vi "GetData.vi"(0 "AlazarCluster":T13, 1 "Digitizer Settings":T9={"Digitizer delay (us) "=0.0, "rf points per line"=2048, "lines per plane"=128, "Samp Rate (Hz)"=100000000.0, "Additional dig delay (us)"=0.0, "Voltage Scale"=0.4, "Pre-Looks"=0, "Offset delay (us)"=0.0, "bits A/D"=8, "Avg Num"=1, "DigTimeOut"=5.0, "Rel Dig Delay"=0.0, "Dig Ch"=0, "LeCroyCluster"={"LeCroy Channels"=[TRUE, FALSE, FALSE, FALSE], "LC read pt offset"=0.0, "Sweep Avg"=FALSE}, "Main Digitizer"=enum."NI Digitizer", "Dig Config"=enum."Single channel", "Digitizer ID Cluster"={"Acqiris/Alazar/SP ID"=[], "NI Instr Handles"=[], "LeCroy VISA"="", "GaGe Handle"={"Handle"=0, "Sample size"=0, "Resolution"=0, "Offset"=0, "Channels"=0, "Boards"=0}, "ATS Ref"="ATS9350", "Acqiris Address"=["PCI::INSTR0"], "ADQRef"=refnum, "adq_cu_ptr"=refnum}, "Trigger Settings"={"Trig Source"=1, "Trig Coupling"=0, "Trig Slope"=0, "Level (mV)"=1500.0}, "Bulk Acq"=FALSE, "Bulk Start Indexes"=[], "Data Ref RF"=refnum, "NI ID/Channel"=[], "Total Dig CH"=1, "Xtra Ann Trig delay (us)"=10.0, "Fix Z Delay?"=FALSE, "One Way Transmission?"=FALSE, "Data Ref Log"=refnum} {"Trigger Settings"."Trig Slope" items=["Positive", "Negative"]; "Trigger Settings"."Level (mV)" format="%.2f"; "Trigger Settings"."Trig Coupling" items=["DC 1 MOhm", "AC 1 MOhm", "DC 50 Ohm", "AC 50 Ohm"]; "Trigger Settings"."Trig Source" items=["Chan 1", "External"]; "Rel Dig Delay" format="%.2f"; "DigTimeOut" format="%.2f"; "Avg Num" min=1; "Offset delay (us)" format="%.2f"; "Additional dig delay (us)" format="%.2f"; "Digitizer delay (us)" format="%.2f"}, 2 "Ann Array Params":T2={"Synth Foc?"=FALSE, "Focal Zones"=41, "Switch T/R"=0, "Trans Geometry (mm)"={"Transducer"=0, "Geo Focus"=12.0, "a (radius)"=3.0, "# of rings"=5, "kerf space "=0.1, "Center Freq"=12.0}, "Sub Ap Excite?"=FALSE, "Full Array Scan?"=FALSE, "Xmt/Rcv"={"XMIT"=[TRUE, TRUE, TRUE, TRUE, TRUE], "RCV"=[TRUE, TRUE, TRUE, TRUE, TRUE]}, "PulseSpacing (us)"=0.0, "Xmit Ring"=0, "XMIT CHS"=0, "RCV CHS"=0, "GPU?"=FALSE, "Save TIFF?"=FALSE, "downfactor"=1, "RCV 1CH"=0} {"RCV 1CH" items=["All", "1", "2", "3", "4", "5"]; "Trans Geometry (mm)"."Transducer" items=["6D 12R 40 MHz"=0, "10D 31R 20 MHz"=1, "10D 23R 20 MHz"=2, "6D 23R 40 MHz"=3, "4.5D 10.7R 40 MHz"=4, "9D 23.5R 20 MHz"=5, "9D 25.8R 20MHz"=6, "Enter"=99]; "Switch T/R" min=1 max=5 step=1}, 3 "Motion Settings":T5={"No Motion?"=FALSE, "Motion System"=enum."NI 735x", "Motion Bd ID"=1, "Motion Profile"="SMAC1", "# Axis"=1, "Reverse Z axis?"=TRUE, "SMAC Axis"=0, "scan pair"=enum."y-(x) scan", "RT fps"=6.0, "Steps per mm"=[1000, 1000, 1000, 1000], "Motor Parameters"={"velocity ct/s"=[10000.0, 10000.0, 10000.0, 50000.0], "accel ct/s^2"=[50000.0, 50000.0, 50000.0, 200000.0]}, "One Way Scan"=FALSE, "Reverse One Way Scan"=FALSE, "Global Position (mm)"=[], "Plane"=0, "Distance between\nscan lines (um)"=0.0, "Distance between\nscan planes (um)"=0.0, "number of scan planes"=1, "Total steps in line"=0, "Xtra plane\ndistance  (um)"=100, "Xtra planes "=1, "Add Axis"=FALSE, "overshoot cts"=200, "BKPT Shift"=0, "Scan Start Time (ms)"=0, "ESP VISA"="GPIB::1::INSTR", "3rd Axis"=1, "GL Ref Out"=refnum, "Galil Address"=""} {"3rd Axis" items=["x", "y", "z", "w"]; "Xtra planes" min=1; "Xtra plane\ndistance  (um)" min=0; "Distance between\nscan planes (um)" format="%.2f"; "Distance between\nscan lines (um)" format="%.2f"; "SMAC Axis" items=["None"=0, "Axis 1"=1, "Axis 2"=2, "Axis 3"=3, "Axis 4"=4, "Axis 5"=5, "Axis 6"=6, "Axis 7"=7, "Axis 8"=8, "Vector Space 1"=17, "Vector Space 2"=18, "Vector Space 3"=19, "Vector Space 4"=20]; "Motion Bd ID" min=1 max=32 step=1}, 4 "All files":string[](array[string]), 5 "error in":errorcluster, 6 "lines per plane mod":i32, 7 "Type of scan":T1, 8 "save?":bool=TRUE, 10 "Start Record":i32, 11 "Reverse ?":bool) -> (12 "Gain Array":T14(array[cluster]), 15 "Raw data out":i16[][][](array[numeric]), 19 "error out":errorcluster)   [LabVIEW 2022 SP3]
uses:
  Digitizers/-DigitizerRoutines/DigitizerSettings.ctl
  Digitizers/-DigitizerRoutines/Digitizer.ctl
  Digitizers/-DigitizerRoutines/DigConfig.ctl
  Digitizers/-DigitizerRoutines/DigitizerID.ctl
  C:/Windows/System32/ADQAPI_dotNet_helper.dll
  Motion Controllers/NI_controller/-NI_MotionRoutines/MotionParameters.ctl
  Motion Controllers/NI_controller/-NI_MotionRoutines/MotionSys.ctl
  Motion Controllers/-MotionRoutines/ScanAxis.ctl
  Motion Controllers/-MotionRoutines/3rdAxis.ctl
  Annular Array/-AnnularRoutines/AnnularArray.ctl
  Annular Array/-AnnularRoutines/TransGeometry.ctl
  Annular Array/-AnnularRoutines/ArrayGeometry.ctl
  Controls/ScanType2.ctl
  Pulsers/PulserGlobals.vi
  Motion Controllers/-MotionRoutines/MotionGlobals.vi
  Digitizers/Acqiris/-AcqirisRoutines/GetAcqSeq.vi
panel:
  # "1-D and 2-D B scan settings"
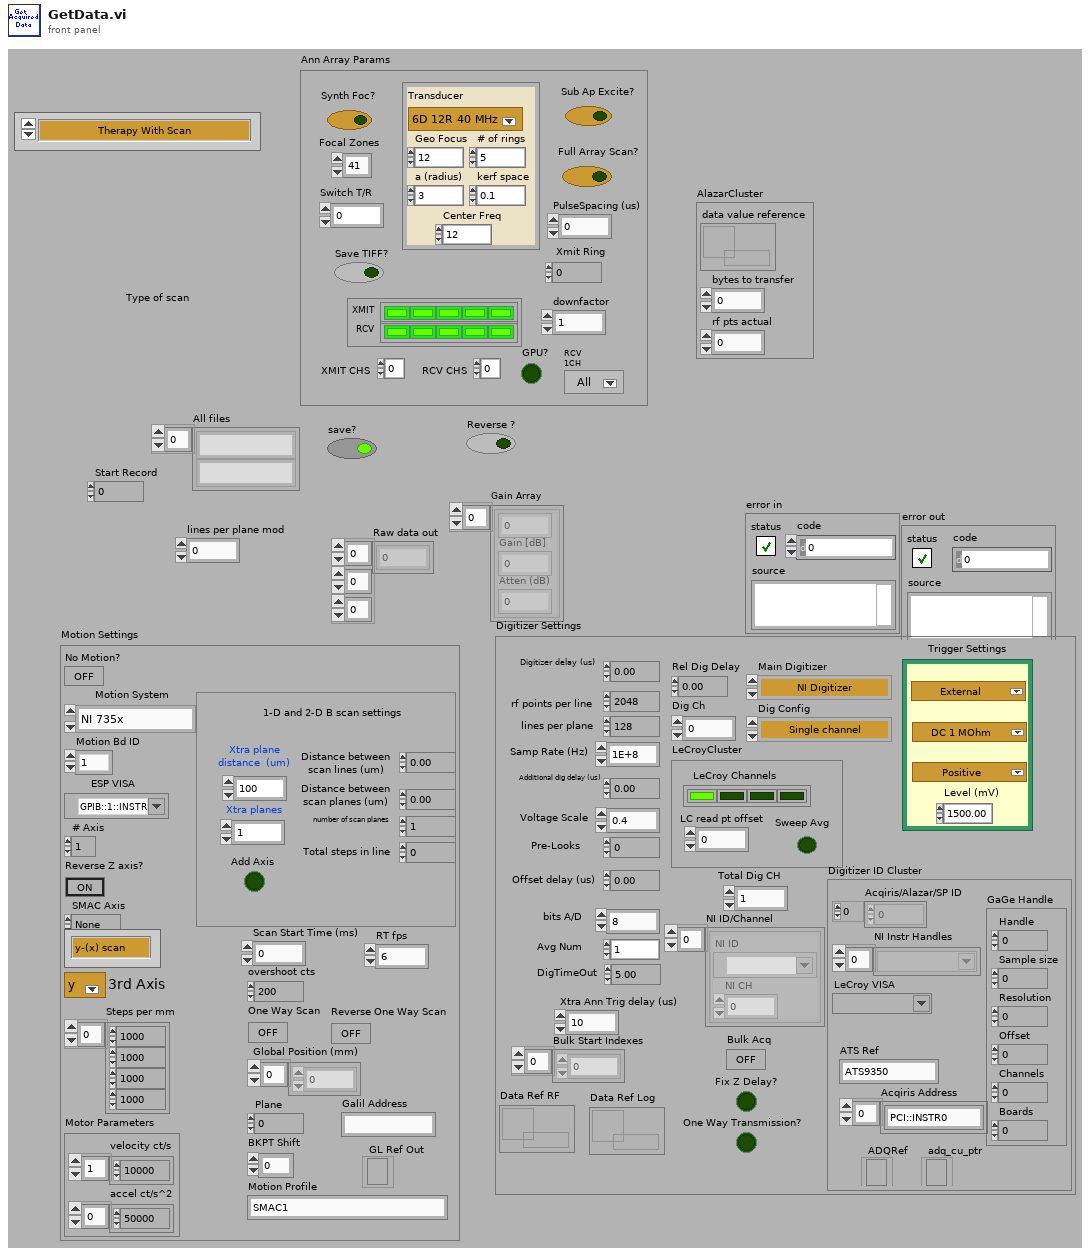
[diagram p1: front panel]
types:
  T1 = typedef "ScanType2.ctl" = enum16{"Therapy With Scan", "M scan", "M Scan With Therapy Burst", "1-D B Scan", "1-D B Scan With Therapy Burst", "2-D B Scan", "2-D B Scan With Therapy Burst", "Rotational Scan", "1-D B-Scan PRF", "2-D B-Scan PRF", "Real-Time Scan", "Contrast Agents", "1-D w/ Real-Time Set Up", "Dual Transducer", "Acoustic Microscopy", "Hydrophone Scanning"}
  T2 = typedef "AnnularArray.ctl" = cluster{"Synth Foc?":bool, "Focal Zones":i16, "Switch T/R":i16, "Trans Geometry (mm)":T3, "Sub Ap Excite?":bool, "Full Array Scan?":bool, "Xmt/Rcv":cluster{"XMIT":bool[], "RCV":bool[]}, "PulseSpacing (us)":sgl, "Xmit Ring":i32, "XMIT CHS":u8, "RCV CHS":u8, "GPU?":bool, "Save TIFF?":bool, "downfactor":i32, "RCV 1CH":u16}
  T3 = typedef "TransGeometry.ctl" = cluster{"Transducer":T4, "Geo Focus":dbl, "a (radius)":dbl, "# of rings":i32, "kerf space ":dbl, "Center Freq":dbl}
  T4 = typedef "ArrayGeometry.ctl" = u16
  T5 = typedef "MotionParameters.ctl" = cluster{"No Motion?":bool, "Motion System":T6, "Motion Bd ID":u8, "Motion Profile":string, "# Axis":i8, "Reverse Z axis?":bool, "SMAC Axis":u16, "scan pair":T7, "RT fps":sgl, "Steps per mm":i32[], "Motor Parameters":cluster{"velocity ct/s":dbl[], "accel ct/s^2":dbl[]}, "One Way Scan":bool, "Reverse One Way Scan":bool, "Global Position (mm)":dbl[], "Plane":i32, "Distance between\nscan lines (um)":sgl, "Distance between\nscan planes (um)":sgl, "number of scan planes":i32, "Total steps in line":i32, "Xtra plane\ndistance  (um)":i32, "Xtra planes ":i32, "Add Axis":bool, "overshoot cts":i32, "BKPT Shift":i32, "Scan Start Time (ms)":u32, "ESP VISA":refnum<visa-resource-name>, "3rd Axis":T8, "GL Ref Out":refnum<k7>, "Galil Address":string}
  T6 = typedef "MotionSys.ctl" = enum16{"MM3000", "NI 735x", "Newport ESP", "No Motion Card", "Galil"}
  T7 = typedef "ScanAxis.ctl" = enum16{"y-(x) scan", "x-(y) scan", "z-(x) scan", "z-(y) scan", "y-(z) scan", "x-(z) scan", "w-(x) scan", "w-(y) scan", "w-(z) scan", "x-(w) scan", "y-(w) scan", "z-(w) scan"}
  T8 = typedef "3rdAxis.ctl" = u16
  T9 = typedef "DigitizerSettings.ctl" = cluster{"Digitizer delay (us) ":dbl, "rf points per line":i32, "lines per plane":i32, "Samp Rate (Hz)":dbl, "Additional dig delay (us)":dbl, "Voltage Scale":dbl, "Pre-Looks":i32, "Offset delay (us)":dbl, "bits A/D":i8, "Avg Num":i32, "DigTimeOut":sgl, "Rel Dig Delay":sgl, "Dig Ch":i32, "LeCroyCluster":cluster{"LeCroy Channels":bool[], "LC read pt offset":dbl, "Sweep Avg":bool}, "Main Digitizer":T10, "Dig Config":T11, "Digitizer ID Cluster":T12, "Trigger Settings":cluster{"Trig Source":u16, "Trig Coupling":u16, "Trig Slope":u16, "Level (mV)":dbl}, "Bulk Acq":bool, "Bulk Start Indexes":i32[], "Data Ref RF":refnum<data-value>, "NI ID/Channel":cluster{"NI ID":refnum<k15>, "NI CH":i32}[], "Total Dig CH":i32, "Xtra Ann Trig delay (us)":dbl, "Fix Z Delay?":bool, "One Way Transmission?":bool, "Data Ref Log":refnum<data-value>}
  T10 = typedef "Digitizer.ctl" = enum16{"Acqiris Digitizer", "NI Digitizer", "LeCroy", "GaGe", "AlazarTech", "No Digitizer", "Teledyne"}
  T11 = typedef "DigConfig.ctl" = enum16{"Single channel", "2 Chans w/ 2 Acqiris", "2 Chans w/ 1 Acqiris", "5-CH Pulser New", "5-CH pulser w/ ann array", "5-pass style ann array", "Empty"}
  T12 = typedef "DigitizerID.ctl" = cluster{"Acqiris/Alazar/SP ID":u32[], "NI Instr Handles":refnum<k15>[], "LeCroy VISA":refnum<visa-resource-name>, "GaGe Handle":cluster{"Handle":u32, "Sample size":u32, "Resolution":i32, "Offset":i32, "Channels":u32, "Boards":u32}, "ATS Ref":string, "Acqiris Address":string[], "ADQRef":refnum<k24>, "adq_cu_ptr":refnum<k24>}
  T13 = cluster{"data value reference":refnum<data-value>, "bytes to transfer":u32, "rf pts actual":u32}
  T14 = cluster{sgl, "Gain [dB]  ":sgl, "Atten (dB)":sgl}[]
  T15 = typedef "NIReadList.ctl" = enum16{"Standard File Dump", "Bulk Acq File Dump", "Send data out", "Synth Focus Each Pass", "Synth Focus Bulk", "5-Ch Pulser File Dump", "5-Ch Pulser Synth Focus", "5-Ch Pulser File Dump AVG"}
  T16 = cluster{sgl, "Gain [dB]  ":sgl, "Atten (dB)":sgl}
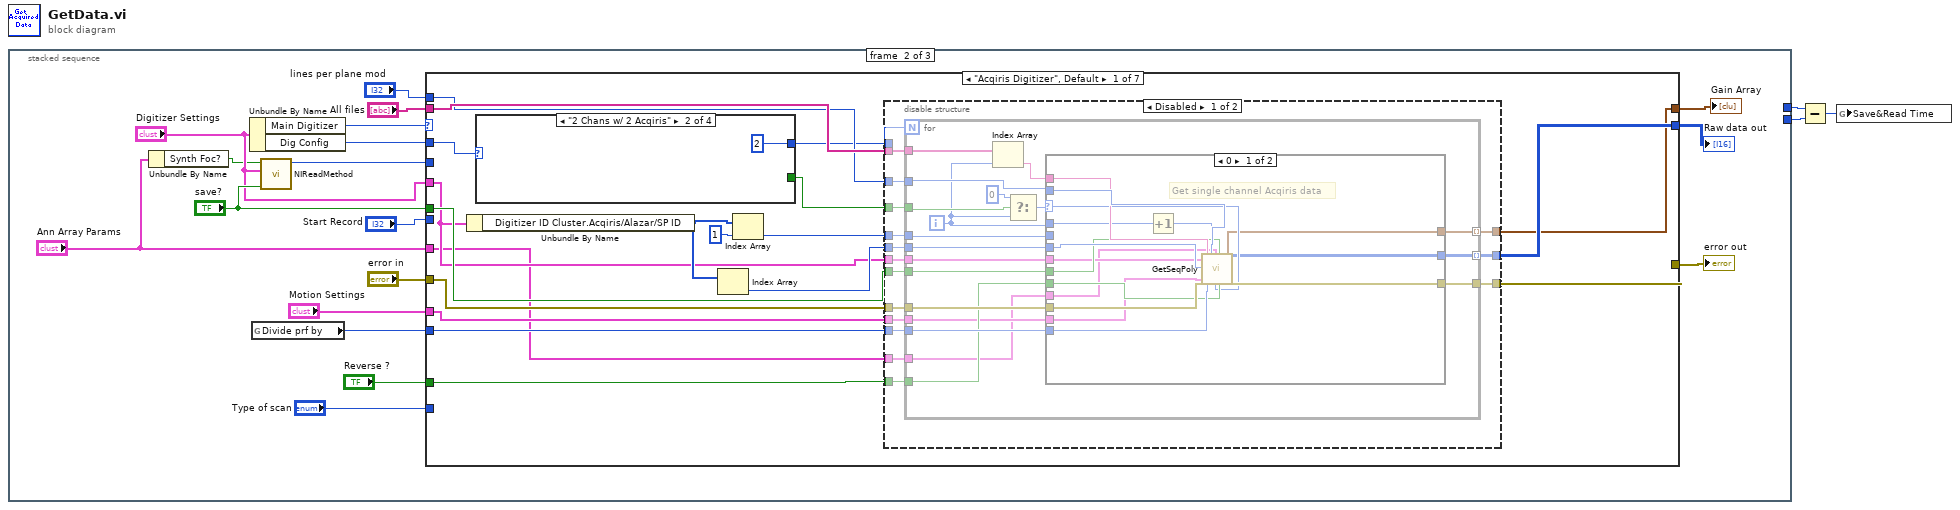
[diagram p0: block diagram]
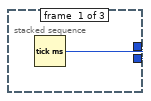
[diagram p2: hidden frame]
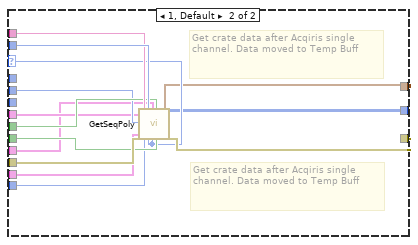
[diagram p3: hidden frame]
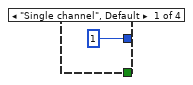
[diagram p5: hidden frame]
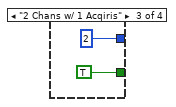
[diagram p6: hidden frame]
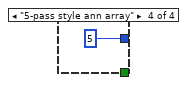
[diagram p7: hidden frame]
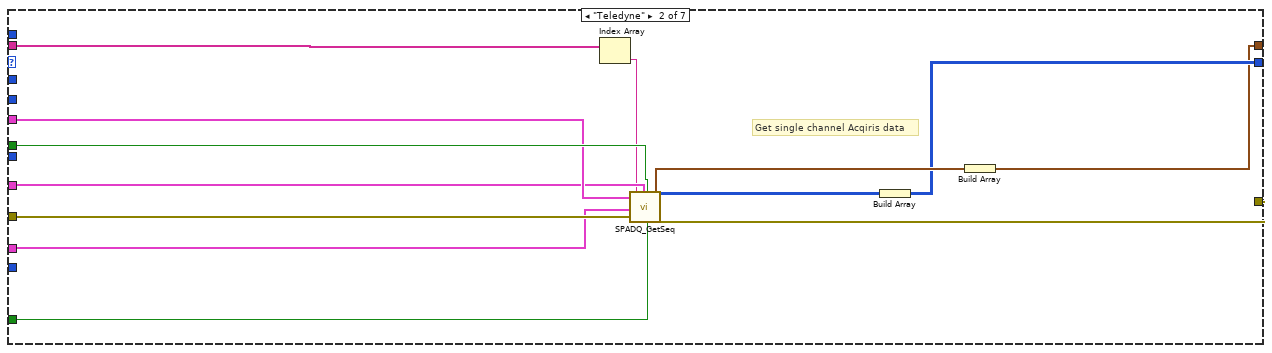
[diagram p8: hidden frame]
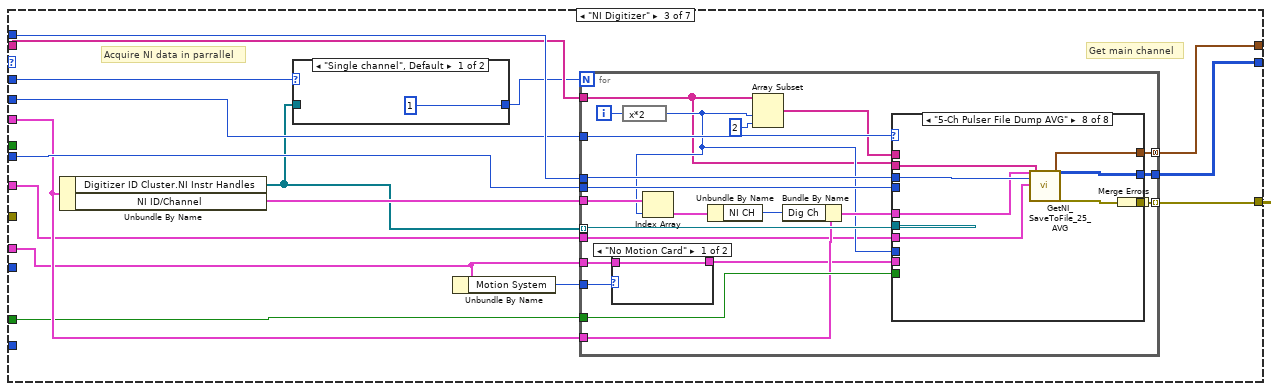
[diagram p9: hidden frame]
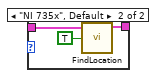
[diagram p10: hidden frame]
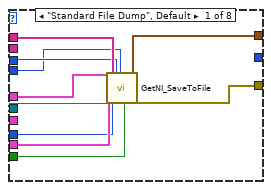
[diagram p11: hidden frame]
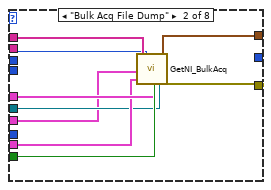
[diagram p12: hidden frame]
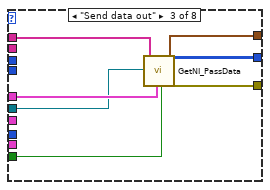
[diagram p13: hidden frame]
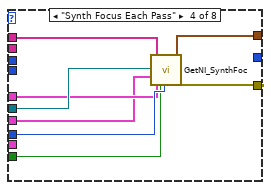
[diagram p14: hidden frame]
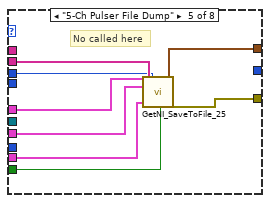
[diagram p15: hidden frame]
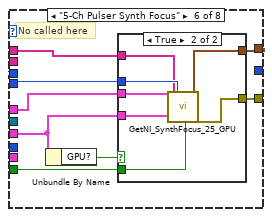
[diagram p16: hidden frame]
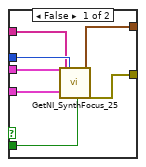
[diagram p17: hidden frame]
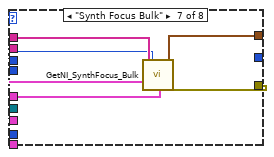
[diagram p18: hidden frame]
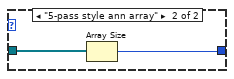
[diagram p19: hidden frame]
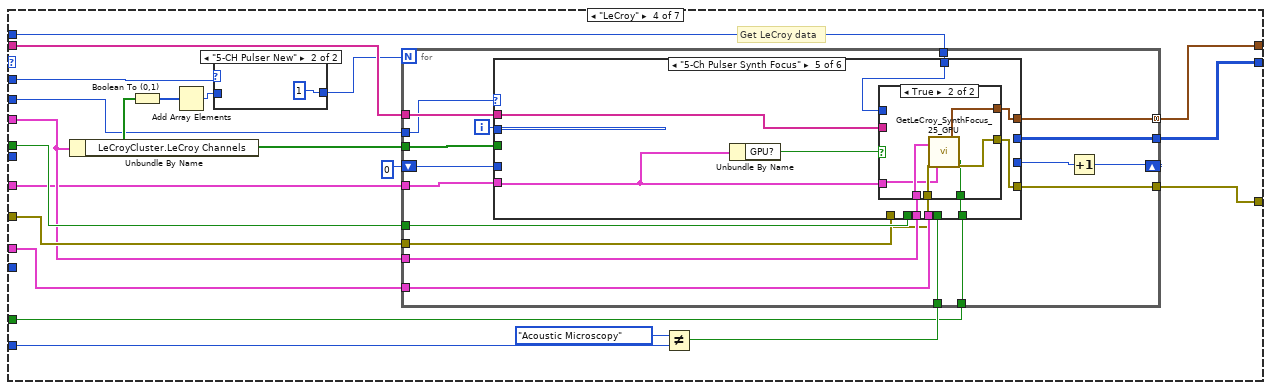
[diagram p20: hidden frame]
diagram:
  n1 = stacked-sequence {
    tunnel: [w4 _ _] -> w2
    tunnel: [_ _ w495] -> w1
    frame #0 {
      n2 = Tick Count (ms)() -> (millisecond timer value=w4:u32)
    }
    frame #1 {
      n3 = Unbundle By Name("Ann Array Params") -> ("Synth Foc?"=w6:bool)
      n4 = Unbundle By Name("Digitizer Settings") -> ("Main Digitizer"=w12:T10, "Dig Config"=w11:T11)
      n5 = global read "PulserGlobals.vi" "Divide prf by"() -> (w8:i32)
      n6 = call "NIReadMethod.vi"("save?"="save?", "Digitizer Settings"="Digitizer Settings", "Synth Foc?"=w6) -> ("Read Method"=w14:T15)  [unwired: 8 in]
      n7 = case shown="\"Acqiris Digitizer\", Default" w12 {
        tunnel: "All files" -> [w41 w124 w137 w259 w388 w413 _]
        tunnel: "Reverse ?" -> [w40 w112 w130 w256 w392 w404 _]
        tunnel: [w39 w123 w141 w249 _ w412 _] -> w20
        tunnel: "lines per plane mod" -> [w38 _ w139 w268 w391 w414 _]
        tunnel: "error in" -> [w37 w122 _ w267 _ w402 _]
        tunnel: w8 -> [w36 _ _ _ _ _ _]
        tunnel: [w35 w114 w132 w248 w383 w416 _] -> w17
        tunnel: "save?" -> [w34 w120 _ w266 w390 _ _]
        tunnel: "Start Record" -> [_ _ w138 _ _ _ _]
        tunnel: w14 -> [_ _ w136 w250 _ w410 _]
        tunnel: w11 -> [w33 _ w134 w255 _ w408 _]
        tunnel: [w30 w113 w129 w251 w384 w411 _] -> w13
        tunnel: "Digitizer Settings" -> [w25 w118 w133 w263 w386 w403 _]
        tunnel: "Motion Settings" -> [w24 w117 w126 w262 w385 w406 _]
        tunnel: "Ann Array Params" -> [w23 w116 w131 w258 _ w405 _]
        tunnel: "Type of scan" -> [_ _ _ w261 _ _ _]
        frame "Acqiris Digitizer", Default {
          n8 = Unbundle By Name(w25) -> ("Digitizer ID Cluster.Acqiris/Alazar/SP ID"=w28:u32[])
          n9 = case shown="\"2 Chans w/ 2 Acqiris\"" w33 {
            tunnel: [1 2 2 5] -> w32
            tunnel: [_ _ TRUE _] -> w31
            frame "Single channel", Default {
            }
            frame "2 Chans w/ 2 Acqiris" {
            }
            frame "2 Chans w/ 1 Acqiris" {
            }
            frame "5-pass style ann array" {
            }
          }
          n10 = Index Array(array=w28) -> (element=w29:u32)  [unwired: 1 in]
          n11 = Index Array(array=w28, index=1) -> (element=w26:u32)
          n12 = disable-structure shown="Disabled" {
            disable-tunnel: w41 -> [w57 _]
            disable-tunnel: w40 -> [w56 _]
            disable-tunnel: [w55 _] -> w39
            disable-tunnel: w38 -> [w54 _]
            disable-tunnel: w37 -> [w53 _]
            disable-tunnel: w36 -> [w52 _]
            disable-tunnel: [w51 _] -> w35
            disable-tunnel: w34 -> [w50 _]
            disable-tunnel: w32 -> [w49 _]
            disable-tunnel: w31 -> [w48 _]
            disable-tunnel: [w47 _] -> w30
            disable-tunnel: w29 -> [w46 _]
            disable-tunnel: w26 -> [w45 _]
            disable-tunnel: w25 -> [w44 _]
            disable-tunnel: w24 -> [w43 _]
            disable-tunnel: w23 -> [w42 _]
            frame Disabled {
              n13 = for {
                N: w49 -> [_]
                tunnel: w52 -> [w76]
                tunnel: w53 -> [w75]
                tunnel: w54 -> [w74]
                tunnel: [w73] -> w55
                tunnel: w56 -> [w72]
                tunnel: w46 -> [w71]
                tunnel: w57 -> [w69]
                tunnel: [w58] -> w51 mode=indexing
                tunnel: w50 -> [w68]
                tunnel: [w67] -> w47 mode=indexing
                tunnel: w48 -> [w66]
                tunnel: w45 -> [w62]
                tunnel: w44 -> [w61]
                tunnel: w43 -> [w60]
                tunnel: w42 -> [w59]
                i -> [w65]
                n14 = Index Array(array=w69, index=w65) -> (element=w70:string)
                n15 = Select(t=0, s=w66, f=w65) -> (s? t:f=w64:i32)
                n16 = case shown="0" w64 {
                  selector: w64 -> [w85 w100]
                  tunnel: w76 -> [w92 w101]
                  tunnel: w75 -> [w91 w106]
                  tunnel: w74 -> [w90 w105]
                  tunnel: [w86 w102] -> w73
                  tunnel: w72 -> [w89 w104]
                  tunnel: w71 -> [w88 _]
                  tunnel: w70 -> [w87 w103]
                  tunnel: [w84 w99] -> w58
                  tunnel: w68 -> [w83 w98]
                  tunnel: [w77 w97] -> w67
                  tunnel: w65 -> [w82 _]
                  tunnel: w62 -> [_ w96]
                  tunnel: w61 -> [w80 w95]
                  tunnel: w60 -> [w79 w94]
                  tunnel: w59 -> [w78 w93]
                  frame 0 {
                    # "Get single channel Acqiris data"
                    n17 = Increment(x=w82) -> (x+1=w81:i32)
                    n18 = call-poly "GetSeqPoly.vi"("Digitizer Settings"=w80, "Acq Card ID"=w88, "Motion Settings"=w79, "errorin"=w91, "Numbered File"=w87, "Divide prf by"=w92, "lines per plane"=w90, "Channel (1)"=w81, "Ann Array Params"=w78, "Rcv Ring"=w85, "save?"=w83, "Reverse?"=w89) -> ("Voltage Scale"=w77:T16, "Array"=w84:i16[][], "error out"=w86:errorcluster)  [unwired: 3 in, 10 out]
                  }
                  frame 1, Default {
                    # "Get crate data after Acqiris single channel. Data moved to Temp Buff"
                    # "Get crate data after Acqiris single channel. Data moved to Temp Buff"
                    n19 = call-poly "GetSeqPoly.vi"("Digitizer Settings"=w95, "Acq Card ID"=w96, "Motion Settings"=w94, "errorin"=w106, "Numbered File"=w103, "Divide prf by"=w101, "lines per plane"=w105, "Channel (1)"=w100, "Ann Array Params"=w93, "Rcv Ring"=w100, "save?"=w98, "Reverse?"=w104) -> ("Voltage Scale"=w97:T16, "Array"=w99:i16[][], "error out"=w102:errorcluster)  [unwired: 3 in, 10 out]
                  }
                }
              }
            }
            frame Enabled {
            }
          }
        }
        frame "Teledyne" {
          # "Get single channel Acqiris data"
          n20 = Index Array(array=w124) -> (element=w115:string)  [unwired: 1 in]
          n21 = call "SPADQ_GetSeq.vi"("Digitizer Settings"=w118, "Motion Settings"=w117, "errorin"=w122, "Numbered File"=w115, "Ann Array Params"=w116, "save?"=w120, "Reverse?"=w112) -> ("Voltage Scale"=w119:T16, "Array"=w121:i16[][], "error out"=w123:errorcluster)  [unwired: 15 in, 3 out]
          n22 = Build Array(w121) -> (w114:i16[][][])
          n23 = Build Array(w119) -> (w113:T14)
        }
        frame "NI Digitizer" {
          # "Acquire NI data in parrallel"
          # "Get main channel"
          n24 = Unbundle By Name(w133) -> ("Digitizer ID Cluster.NI Instr Handles"=w127:refnum<k15>[], "NI ID/Channel"=w135:cluster{"NI ID":refnum<k15>, "NI CH":i32}[])
          n25 = case shown="\"Single channel\", Default" w134 {
            tunnel: w127 -> [_ w247]
            tunnel: [1 ("Rcv Ring") w246] -> w128
            frame "Single channel", Default {
            }
            frame "5-pass style ann array" {
              n26 = Array Size(array=w247) -> (size(s)=w246:i32)
            }
          }
          n27 = Unbundle By Name(w126) -> ("Motion System"=w125:T6)
          n28 = for {
            N: w128 -> [_]
            tunnel: [w163] -> w129 mode=concatenating
            tunnel: [w162] -> w132
            tunnel: [w161] -> w140 mode=indexing
            tunnel: w136 -> [w160]
            tunnel: w138 -> [w159]
            tunnel: w139 -> [w158]
            tunnel: w130 -> [w157]
            tunnel: w133 -> [w150]
            tunnel: w126 -> [w146]
            tunnel: w127 -> [w156] mode=indexing
            tunnel: w137 -> [w143]
            tunnel: w135 -> [w153]
            tunnel: w131 -> [w147]
            tunnel: w125 -> [w142]
            i -> [w155]
            n29 = case shown="\"No Motion Card\"" w142 {
              tunnel: w146 -> [w164 w167]
              tunnel: [w164 w166] -> w145
              frame "No Motion Card" {
              }
              frame "NI 735x", Default {
                n30 = call "FindLocation.vi"("Motion Settings"=w167, "Wait for Motion Complete"=TRUE) -> ("Motion Settings Out"=w166:T5)  [unwired: 1 in, 3 out]
              }
            }
            n31 = expression code="x*2"(w155) -> (w148:i32)
            n32 = Index Array(array=w153, index=w148) -> (element=w152:cluster{"NI ID":refnum<k15>, "NI CH":i32})
            n33 = Unbundle By Name(w152) -> ("NI CH"=w151:i32)
            n34 = Array Subset(array=w143, index=w148, length=2) -> (w144:string[])
            n35 = Bundle By Name(cluster=w150, "Dig Ch"=w151) -> (w149:T9)
            n36 = case shown="\"5-Ch Pulser File Dump AVG\"" w160 {
              tunnel: [w177 w186 w193 w201 w209 w217 w237 w243] -> w163
              tunnel: w144 -> [w176 w185 w192 w200 _ w215 w236 _]
              tunnel: [_ _ w189 _ _ _ _ w244] -> w162
              tunnel: [w175 w184 w191 w199 w208 w214 w233 w242] -> w161
              tunnel: w157 -> [w168 w183 w190 w194 w203 w212 _ _]
              tunnel: w158 -> [w174 w182 _ _ w204 w216 w234 w241]
              tunnel: w159 -> [w173 _ _ _ _ _ _ _]
              tunnel: w148 -> [w170 _ _ w198 _ _ _ _]
              tunnel: w149 -> [w172 w181 w188 w196 w206 w210 w235 w239]
              tunnel: w145 -> [w171 w180 _ _ w205 _ _ _]
              tunnel: w156 -> [w169 w179 w187 w197 _ _ _ _]
              tunnel: w143 -> [_ _ _ _ w207 _ _ w240]
              tunnel: w147 -> [_ w178 _ w195 w202 w211 w232 w238]
              frame "Standard File Dump", Default {
                n37 = call "GetNI_SaveToFile.vi"("Digitizer Settings"=w172, "NI Card"=w169, "Motion Settings"=w171, "File Array"=w176, "Pulser Channel"=w170, "lines per plane"=w174, "Start Record"=w173, "Reverse?"=w168) -> ("Gain Array"=w177:T14, "error out"=w175:errorcluster)  [unwired: 16 in, 2 out]
              }
              frame "Bulk Acq File Dump" {
                n38 = call "GetNI_BulkAcq.vi"("Digitizer Settings"=w181, "NI Card"=w179, "Ann Array Params"=w178, "Motion Settings"=w180, "File Array"=w185, "lines per plane"=w182, "Reverse?"=w183) -> ("Gain Array"=w186:T14, "error out"=w184:errorcluster)  [unwired: 17 in, 2 out]
              }
              frame "Send data out" {
                n39 = call "GetNI_PassData.vi"("Digitizer Settings"=w188, "NI Card"=w187, "File Array"=w192, "Reverse?"=w190) -> ("Gain Array"=w193:T14, "Array"=w189:i16[][][], "error out"=w191:errorcluster)  [unwired: 19 in, 2 out]
              }
              frame "Synth Focus Each Pass" {
                n40 = call "GetNI_SynthFoc.vi"("Digitizer Settings"=w196, "NI Card"=w197, "Ann Array Params"=w195, "File Array"=w200, "Reverse ?"=w194, "Rcv Ring"=w198) -> ("Gain Array"=w201:T14, "error out"=w199:errorcluster)  [unwired: 17 in, 3 out]
              }
              frame "5-Ch Pulser File Dump" {
                # "No called here"
                n41 = call "GetNI_SaveToFile_25.vi"("Digitizer Settings"=w206, "Ann Array Params"=w202, "Motion Settings"=w205, "File Array"=w207, "lines per plane"=w204, "Reverse?"=w203) -> ("Gain Array"=w209:T14, "error out"=w208:errorcluster)  [unwired: 18 in, 2 out]
              }
              frame "5-Ch Pulser Synth Focus" {
                # "No called here"
                n42 = Unbundle By Name(w211) -> ("GPU?"=w213:bool)
                n43 = case shown="True" w213 {
                  tunnel: [w224 w230] -> w217
                  tunnel: w216 -> [w223 w229]
                  tunnel: w215 -> [w222 w228]
                  tunnel: w210 -> [w221 w227]
                  tunnel: [w220 w231] -> w214
                  tunnel: w211 -> [w219 w226]
                  tunnel: w212 -> [w218 w225]
                  frame False {
                    n44 = call "GetNI_SynthFocus_25.vi"("Digitizer Settings"=w221, "File Array"=w222, "Ann Array Params"=w219, "lines per plane"=w223, "Reverse?"=w218) -> ("Gain Array"=w224:T14, "error out"=w220:errorcluster)  [unwired: 19 in, 2 out]
                  }
                  frame True {
                    n45 = call "GetNI_SynthFocus_25_GPU.vi"("Digitizer Settings"=w227, "File Array"=w228, "Ann Array Params"=w226, "lines per plane"=w229, "Reverse?"=w225) -> ("Gain Array"=w230:T14, "error out"=w231:errorcluster)  [unwired: 19 in, 2 out]
                  }
                }
              }
              frame "Synth Focus Bulk" {
                n46 = call "GetNI_SynthFocus_Bulk.vi"("Digitizer Settings"=w235, "Ann Array Params"=w232, "File Array"=w236, "lines per plane"=w234) -> ("Gain Array"=w237:T14, "error out"=w233:errorcluster)  [unwired: 20 in, 2 out]
              }
              frame "5-Ch Pulser File Dump AVG" {
                n47 = call "GetNI_SaveToFile_25_AVG.vi"("Digitizer Settings"=w239, "Ann Array Params"=w238, "File Array"=w240, "lines per plane"=w241) -> ("Gain Array"=w243:T14, "data out"=w244:i8[][][], "error out"=w242:errorcluster)  [unwired: 19 in, 2 out]
              }
            }
          }
          n48 = Merge Errors(w140) -> (w141:errorcluster)
        }
        frame "LeCroy" {
          # "Get LeCroy data"
          n49 = Unbundle By Name(w263) -> ("LeCroyCluster.LeCroy Channels"=w252:bool[])
          n50 = Boolean To (0,1)(Boolean=w252) -> (0, 1=w265:i16[])
          n51 = Add Array Elements(numeric array=w265) -> (sum=w254:i16)
          n52 = case shown="\"5-CH Pulser New\"" w255 {
            tunnel: [w269 1] -> w253
            tunnel: w254 -> [w269 _]
            frame "Single channel", Default {
            }
            frame "5-CH Pulser New" {
            }
          }
          n53 = Not Equal?(x=ScanType2."Acoustic Microscopy", y=w261) -> (x != y?=w257:bool)
          n54 = for {
            N: w253 -> [_]
            tunnel: w267 -> [w278]
            tunnel: w268 -> [w282]
            tunnel: [w275] -> w249
            tunnel: [w276] -> w248
            tunnel: w266 -> [w281]
            tunnel: [w277] -> w251 mode=concatenating
            tunnel: w252 -> [w274]
            shift-right: [w288] -> _
            shift-left: 0 -> [w273]
            tunnel: w263 -> [w284]
            tunnel: w262 -> [w283]
            tunnel: w259 -> [w286]
            tunnel: w258 -> [w285]
            tunnel: w257 -> [w280]
            tunnel: w256 -> [w279]
            tunnel: w250 -> [w271]
            i -> [w287]
            n55 = case shown="\"5-Ch Pulser Synth Focus\"" w271 {
              tunnel: w287 -> [w305 _ w337 _ _ _]
              tunnel: w286 -> [w304 w314 w336 w353 w361 w379]
              tunnel: w285 -> [_ _ w335 w349 w355 _]
              tunnel: w284 -> [w298 w315 w332 w348 w360 w380]
              tunnel: w283 -> [w300 _ w331 w347 _ _]
              tunnel: w282 -> [_ w313 _ w345 w362 w378]
              tunnel: w281 -> [w301 _ w330 _ _ _]
              tunnel: w280 -> [w297 _ w329 _ _ _]
              tunnel: w279 -> [w302 w316 w328 w346 w354 _]
              tunnel: w278 -> [w299 _ w327 w350 w359 _]
              tunnel: [w290 w318 w320 w352 w358 w382] -> w277
              tunnel: [_ w319 _ _ _ w377] -> w276
              tunnel: [w296 w317 w325 w351 w357 w381] -> w275
              tunnel: w274 -> [w294 _ w323 _ _ _]
              tunnel: w273 -> [w292 _ w322 _ _ _]
              tunnel: [w291 _ w321 _ _ _] -> w272
              frame "Standard File Dump", Default {
                n56 = Search 1D Array(1D array=w294, element=TRUE, start index (0)=w292) -> (index of element=w291:i32)
                n57 = Index Array(array=w304) -> (element=w303:string)  [unwired: 1 in]
                n58 = case shown="1, Default" w305 {
                  tunnel: w303 -> [w306 w312]
                  tunnel: [w306 w309] -> w295
                  tunnel: w291 -> [_ w307]
                  frame 0 {
                  }
                  frame 1, Default {
                    n59 = Increment(x=w307) -> (x+1=w308:i32)
                    n60 = Number To Decimal String(number=w308) -> (decimal integer string=w310:string)  [unwired: 1 in]
                    n61 = Concatenate Strings(w312, "_CH" ("string"), w310) -> (w309:string)
                  }
                }
                n62 = call "GetAcqSeqLeCroy.vi"("Digitizer Settings"=w298, "Motion Settings"=w300, "errorin"=w299, "Numbered File"=w295, "Pop Up"=w297, "Source (0: Channel 1)"=w291, "save?"=w301, "Reverse?"=w302) -> ("Voltage Scale"=w289:T16, "error out"=w296:errorcluster)  [unwired: 13 in, 5 out]
                n63 = Build Array(w289) -> (w290:T14)
              }
              frame "Send data out" {
                n64 = call "GetLeCroy_PassData.vi"("lines per plane"=w313, "File Array"=w314, "Digitizer Settings"=w315, "Reverse?"=w316) -> ("Gain Array"=w318:T14, "Array out"=w319:i16[][][], "error out"=w317:errorcluster)  [unwired: 7 in, 2 out]
              }
              frame "Bulk Acq File Dump" {
                n65 = Unbundle By Name(w335) -> ("RCV 1CH"=w334:u16)
                n66 = Search 1D Array(1D array=w323, element=TRUE, start index (0)=w322) -> (index of element=w321:i32)
                n67 = case shown="0" w334 {
                  selector: w334 -> [_ w342]
                  tunnel: [w340 w343] -> w333
                  tunnel: w337 -> [w339 _]
                  tunnel: w336 -> [w338 w344]
                  frame 0 {
                    n68 = Index Array(array=w338, index=w339) -> (element=w340:string)
                  }
                  frame 1, Default {
                    n69 = Decrement(x=w342) -> (x-1=w341:u16)
                    n70 = Index Array(array=w344, index=w341) -> (element=w343:string)
                  }
                }
                n71 = call "GetAcqSeqLeCroy.vi"("Digitizer Settings"=w332, "Motion Settings"=w331, "errorin"=w327, "Numbered File"=w333, "Pop Up"=w329, "Source (0: Channel 1)"=w321, "save?"=w330, "Reverse?"=w328) -> ("Voltage Scale"=w326:T16, "error out"=w325:errorcluster)  [unwired: 13 in, 5 out]
                n72 = Build Array(w326) -> (w320:T14)
              }
              frame "5-Ch Pulser File Dump" {
                n73 = call "GetLeCroy_SaveToFile_25.vi"("Digitizer Settings"=w348, "Ann Array Params"=w349, "errorin"=w350, "File Array"=w353, "Motion Settings"=w347, "lines per plane"=w345, "Reverse?"=w346) -> ("Gain Array"=w352:T14, "error out"=w351:errorcluster)  [unwired: 9 in, 2 out]
              }
              frame "5-Ch Pulser Synth Focus" {
                n74 = Unbundle By Name(w355) -> ("GPU?"=w356:bool)
                n75 = case shown="True" w356 {
                  tunnel: [w370 w376] -> w357
                  tunnel: [w369 w375] -> w358
                  tunnel: w362 -> [w368 _]
                  tunnel: w361 -> [w367 _]
                  tunnel: w354 -> [w363 w371]
                  tunnel: w360 -> [w366 w374]
                  tunnel: w359 -> [w365 w373]
                  tunnel: w355 -> [w364 w372]
                  frame False {
                    n76 = call "GetLeCroy_SynthFocus_25.vi"("Digitizer Settings"=w366, "errorin"=w365, "File Array"=w367, "Ann Array Params"=w364, "lines per plane"=w368, "Reverse?"=w363) -> ("Gain Array"=w369:T14, "error out"=w370:errorcluster)  [unwired: 10 in, 2 out]
                  }
                  frame True {
                    n77 = call "GetLeCroy_SynthFocus_25_GPU.vi"("Digitizer Settings"=w374, "errorin"=w373, "Ann Array Params"=w372, "Reverse?"=w371) -> ("Gain Array"=w375:T14, "error out"=w376:errorcluster)  [unwired: 12 in, 2 out]
                  }
                }
              }
              frame "5-Ch Pulser File Dump AVG" {
                n78 = call "GetLeCroy_SaveToFile_25_AVG.vi"("File Array"=w379, "lines per plane"=w378, "Digitizer Settings"=w380) -> ("Gain Array"=w382:T14, "data out"=w377:i16[][][], "error out"=w381:errorcluster)  [unwired: 8 in, 2 out]
              }
            }
            n79 = Increment(x=w272) -> (x+1=w288:i32)
          }
        }
        frame "GaGe" {
          # "Get single channel Gage data"
          n80 = Index Array(array=w388) -> (element=w387:string)  [unwired: 1 in]
          n81 = for {
            N: 1 -> [_]
            tunnel: w391 -> [w401]
            tunnel: w392 -> [w400]
            tunnel: [w399] -> w383 mode=indexing
            tunnel: w390 -> [w398]
            tunnel: [w397] -> w384 mode=indexing
            tunnel: w387 -> [w395]
            tunnel: w386 -> [w394]
            tunnel: w385 -> [w393]
            i -> [w396]
            n82 = call "GetAcqSeqGageFill.vi"("Digitizer Settings"=w394, "Motion Settings 2"=w393, "Numbered File"=w395, "lines per plane"=w401, "Channel"=w396, "save?"=w398, "Reverse?"=w400) -> ("Voltage Scale"=w397:T16, "Array"=w399:i16[][])  [unwired: 17 in, 2 out]
          }
        }
        frame "AlazarTech" {
          # "Pass on data"
          # "Acquire Alazar data in parrallel"
          # "Get main channel"
          n83 = case shown="\"5-CH Pulser New\", \"5-CH pulser w/ ann array\"" w408 {
            tunnel: [1 4] -> w407
            frame "Single channel", Default {
            }
            frame "5-CH Pulser New", "5-CH pulser w/ ann array" {
            }
          }
          n84 = Array Subset(array=w413, length=w407) -> (w415:string[])  [unwired: 1 in]
          n85 = case shown="\"5-Ch Pulser File Dump AVG\"" w410 {
            tunnel: [w428 w437 w448 w457 w467 w493] -> w411
            tunnel: w415 -> [w420 w430 w444 _ _ _]
            tunnel: [_ w436 w447 _ _ w492] -> w416
            tunnel: [w427 w435 w446 w458 w468 w494] -> w412
            tunnel: w404 -> [w425 w434 w439 w449 w463 _]
            tunnel: w414 -> [w421 w432 w443 w455 w466 w491]
            tunnel: w413 -> [_ _ _ w454 w465 w489]
            tunnel: "AlazarCluster" -> [w422 w431 w442 w456 w464 w490]
            tunnel: w403 -> [w424 w429 w441 w450 w462 w488]
            tunnel: w406 -> [w426 _ _ w452 _ _]
            tunnel: w405 -> [w423 _ w440 w451 w460 w486]
            tunnel: w402 -> [w419 w433 w438 w453 w461 w487]
            frame "Standard File Dump", Default {
              n86 = call "GetAlazar_SaveToFile - ATS-SDK.vi"("File Array"=w420, "lines per plane"=w421, "Digitizer Settings"=w424, "Ann Array Params"=w423, "AlazarCluster"=w422, "errorin"=w419, "Motion Settings"=w426, "Reverse?"=w425) -> ("Gain Array"=w428:T14, "error out"=w427:errorcluster)  [unwired: 4 in, 2 out]
            }
            frame "Send data out" {
              n87 = call "GetAlazar_PassData - ATS-SDK.vi"("lines per plane"=w432, "File Array"=w430, "Digitizer Settings"=w429, "AlazarCluster"=w431, "error in"=w433, "Reverse?"=w434) -> ("Gain Array"=w437:T14, "Array out"=w436:i16[][][], "error out"=w435:errorcluster)  [unwired: 5 in, 2 out]
            }
            frame "Synth Focus Each Pass" {
              n88 = call "GetAlazar_SynthFoc - ATS-SDK.vi"("Digitizer Settings"=w441, "AlazarCluster"=w442, "Reverse ?"=w439, "errorin"=w438, "File Array"=w444, "Ann Array Params"=w440, "lines per plane"=w443, "Rcv Ring"=0) -> ("Gain Array"=w448:T14, "Array out"=w447:i16[][][], "error out"=w446:errorcluster)  [unwired: 7 in, 2 out]
            }
            frame "5-Ch Pulser File Dump" {
              n89 = call "GetAlazar_SaveToFile_25 - ATS-SDK.vi"("Digitizer Settings"=w450, "AlazarCluster"=w456, "Ann Array Params"=w451, "errorin"=w453, "File Array"=w454, "Motion Settings"=w452, "lines per plane"=w455, "Reverse?"=w449) -> ("Gain Array"=w457:T14, "error out"=w458:errorcluster)  [unwired: 8 in, 2 out]
            }
            frame "5-Ch Pulser Synth Focus" {
              n90 = Unbundle By Name(w460) -> ("GPU?"=w459:bool)
              n91 = case shown="False" w459 {
                tunnel: [w477 w485] -> w468
                tunnel: [w476 w484] -> w467
                tunnel: w466 -> [w475 w483]
                tunnel: w465 -> [w474 _]
                tunnel: w464 -> [w469 w482]
                tunnel: w463 -> [w473 w481]
                tunnel: w460 -> [w472 w480]
                tunnel: w462 -> [w471 w479]
                tunnel: w461 -> [w470 w478]
                frame False {
                  n92 = call "GetAlazar_SynthFocus_25 - ATS-SDK.vi"("Digitizer Settings"=w471, "AlazarCluster"=w469, "errorin"=w470, "File Array"=w474, "Ann Array Params"=w472, "lines per plane"=w475, "Reverse?"=w473) -> ("Gain Array"=w476:T14, "error out"=w477:errorcluster)  [unwired: 9 in, 2 out]
                }
                frame True {
                  n93 = call "GetAlazar_SynthFocus_25_GPU - ATS-SDK.vi"("Digitizer Settings"=w479, "AlazarCluster"=w482, "errorin"=w478, "Ann Array Params"=w480, "lines per plane"=w483, "Reverse?"=w481) -> ("Gain Array"=w484:T14, "error out"=w485:errorcluster)  [unwired: 10 in, 2 out]
                }
              }
            }
            frame "5-Ch Pulser File Dump AVG" {
              n94 = call "GetAlazar_SaveToFile_25_AVG - ATS-SDK.vi"("File Array"=w489, "lines per plane"=w491, "Digitizer Settings"=w488, "AlazarCluster"=w490, "Ann Array Params"=w486, "errorin"=w487) -> ("Gain Array"=w493:T14, "data out"=w492:i16[][][], "error out"=w494:errorcluster)  [unwired: 5 in, 2 out]
            }
          }
        }
        frame "No Digitizer" {
        }
      }
      "error out" <- w20
      "Raw data out" <- w17
      "Gain Array" <- w13
    }
    frame #2 {
      # "Capture time of subroutine"
      n95 = Tick Count (ms)() -> (millisecond timer value=w495:u32)
    }
  }
  n96 = Subtract(x=w1, y=w2) -> (x-y=w3:u32)
  n97 = global write "MotionGlobals.vi" "Save&Read Time"(w3) -> ()
